vi "Set_AutoSet_ExposureTime.vi"(8 "error in (no error)":errorcluster, 9 "Max. ExposureTime":dbl[unit], 10 "Maximal counts":dbl=65000.0, 11 "Abstract_CCD in":refnum<class "Abstract_CCD.lvclass">) -> (0 "error out":errorcluster, 3 "Abstract_CCD out":refnum<class "Abstract_CCD.lvclass">)   [LabVIEW 2020, in "Abstract_CCD.lvclass"]
uses:
  <instrlib>/Classes/CCD/Abstract_CCD/Abstract_CCD.lvclass
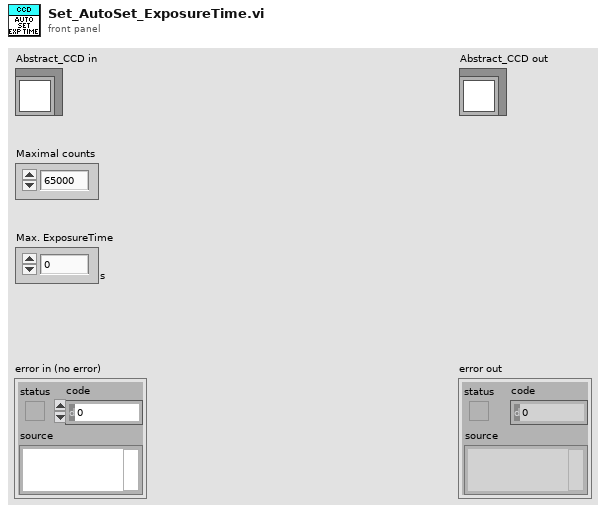
[diagram p1: front panel]
types:
  T1 = cluster{"Image":dbl[][][], "Frame Size":cluster{"F":i32, "Y":i32, "X":i32}}[]
  T2 = cluster{"Image":dbl[][][], "Frame Size":cluster{"F":i32, "Y":i32, "X":i32}}
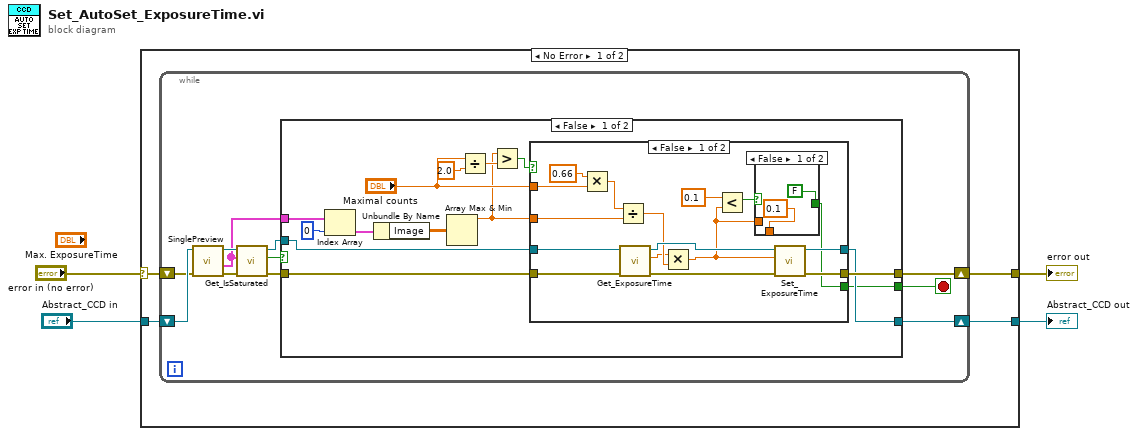
[diagram p0: block diagram]
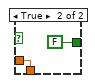
[diagram p2: hidden frame]
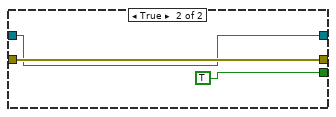
[diagram p3: hidden frame]
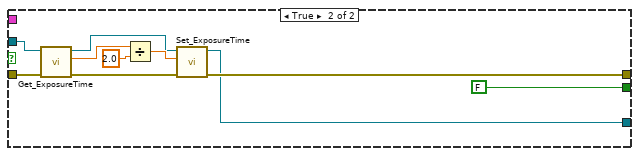
[diagram p4: hidden frame]
diagram:
  n1 = case shown="No Error" "error in (no error)" {
    selector: "error in (no error)" -> [w8 w68]
    tunnel: [w5 w68] -> w3
    tunnel: [w6 w67] -> w1
    tunnel: "Abstract_CCD in" -> [w7 w67]
    frame No Error {
      n2 = while {
        shift-right: [w10] -> w6
        shift-left: w7 -> [w19]
        shift-right: [w11] -> w5
        shift-left: w8 -> [w18]
        stop <- w9 stop-if-true
        n3 = call-dynamic "SinglePreview.vi"("error in (no error)"=w18, "Abstract_CCD in"=w19) -> ("error out"=w17:errorcluster, "Data Raw"=w12:T1, "Abstract_CCD out"=w16:refnum<class "Abstract_CCD.lvclass">)  [unwired: 5 in, 2 out]
        n4 = call-dynamic "Get_IsSaturated.vi"("error in (no error)"=w17, "Data Raw"=w12, "Abstract_CCD in"=w16) -> ("error out"=w14:errorcluster, "Is Saturated?"=w15:bool, "Abstract_CCD out"=w13:refnum<class "Abstract_CCD.lvclass">)  [unwired: 6 in]
        n5 = case shown="False" w15 {
          tunnel: w14 -> [w26 w62]
          tunnel: w13 -> [w24 w61]
          tunnel: w12 -> [w33 _]
          tunnel: [w25 w59] -> w11
          tunnel: [w23 w58] -> w10
          tunnel: [w22 FALSE] -> w9
          frame False {
            n6 = Index Array(array=w33, index=0) -> (element=w31:T2)
            n7 = Unbundle By Name(w31) -> ("Image"=w30:dbl[][][])
            n8 = Array Max & Min(array=w30) -> (max value=w20:dbl)  [unwired: 3 out]
            n9 = Divide(x="Maximal counts", y=2.0) -> (x/y=w28:dbl)
            n10 = Greater?(x=w20, y=w28) -> (0:w27:bool)
            n11 = case shown="False" w27 {
              tunnel: w26 -> [w48 w56]
              tunnel: [w45 w56] -> w25
              tunnel: w24 -> [w49 w55]
              tunnel: [w44 w55] -> w23
              tunnel: [w35 TRUE] -> w22
              tunnel: "Maximal counts" -> [w42 _]
              tunnel: w20 -> [w43 _]
              frame False {
                n12 = Multiply(x=0.66, y=w42) -> (x*y=w40:dbl)
                n13 = Divide(x=w40, y=w43) -> (x/y=w39:dbl)
                n14 = call-dynamic "Get_ExposureTime.vi"("error in (no error)"=w48, "Abstract_CCD in"=w49) -> ("error out"=w47:errorcluster, "Exposure Time"=w38:dbl[unit], "Abstract_CCD out"=w46:refnum<class "Abstract_CCD.lvclass">)  [unwired: 7 in]
                n15 = Multiply(x=w38, y=w39) -> (x*y=w34:dbl[unit])
                n16 = Less?(x=dbl[unit] 0.1, y=w34) -> (x < y?=w36:bool)
                n17 = case shown="False" w36 {
                  tunnel: [dbl[unit] 0.1 ("x") w53] -> _
                  tunnel: w34 -> [_ w53]
                  tunnel: [FALSE FALSE] -> w35
                  frame False {
                  }
                  frame True {
                  }
                }
                n18 = call-dynamic "Set_ExposureTime.vi"("error in (no error)"=w47, "Exposure Time"=w34, "Abstract_CCD in"=w46) -> ("error out"=w45:errorcluster, "Abstract_CCD out"=w44:refnum<class "Abstract_CCD.lvclass">)  [unwired: 7 in]
              }
              frame True {
              }
            }
          }
          frame True {
            n19 = call-dynamic "Get_ExposureTime.vi"("error in (no error)"=w62, "Abstract_CCD in"=w61) -> ("error out"=w60:errorcluster, "Exposure Time"=w66:dbl[unit], "Abstract_CCD out"=w63:refnum<class "Abstract_CCD.lvclass">)  [unwired: 7 in]
            n20 = Divide(x=w66, y=2.0) -> (x/y=w64:dbl[unit])
            n21 = call-dynamic "Set_ExposureTime.vi"("error in (no error)"=w60, "Exposure Time"=w64, "Abstract_CCD in"=w63) -> ("error out"=w59:errorcluster, "Abstract_CCD out"=w58:refnum<class "Abstract_CCD.lvclass">)  [unwired: 7 in]
          }
        }
      }
    }
    frame Error {
    }
  }
  "error out" <- w3
  "Abstract_CCD out" <- w1
